vi "box.vi"(8 "error in (no error)":errorcluster, 11 "node":refnum<data-value>) -> (0 "error out":errorcluster, 3 "DoublyNodeRef out":refnum<class "DoublyNodeRef.lvclass">)   [LabVIEW 2021, in "DoublyNodeRef.lvclass"]
uses:
  DoublyNodeRef.lvclass
  IDoublyNode/IDoublyNode.lvclass
  DoublyNodeRef.lvclass/DoublyNodeRef.ctl
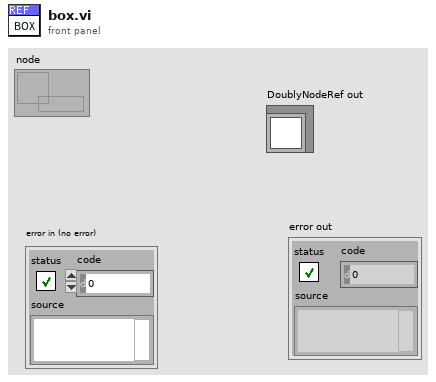
[diagram p1: front panel]
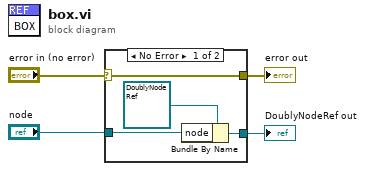
[diagram p0: block diagram]
diagram:
  n1 = case shown="No Error" "error in (no error)" {
    selector: "error in (no error)" -> [w8 w9]
    tunnel: [w8 w9] -> w3
    tunnel: [w7 _] -> w2
    tunnel: "node" -> [w6 _]
    frame No Error {
      n2 = Bundle By Name(cluster=refnum<class "DoublyNodeRef.lvclass"> refnum ("DoublyNodeRef in"), "node"=w6) -> (w7:refnum<class "DoublyNodeRef.lvclass">)
    }
    frame Error {
    }
  }
  "error out" <- w3
  "DoublyNodeRef out" <- w2
